vi "LPF.vi"(9 "Cutoff freq":dbl, 10 "Sampling freq":dbl, 11 "x":dbl) -> (2 "y":dbl)   [LabVIEW 2025]
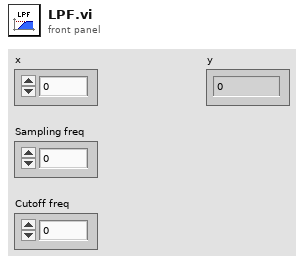
[diagram p1: front panel]
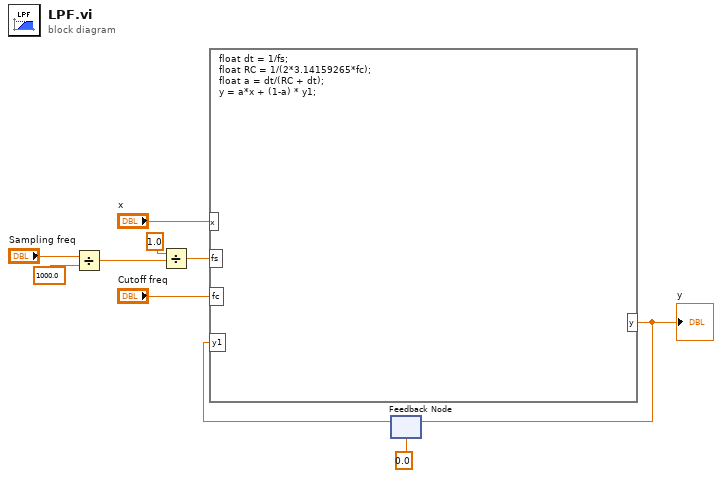
[diagram p0: block diagram]
diagram:
  n1 = Divide(x="Sampling freq", y=1000.0) -> (x/y=w3:dbl)
  n2 = Divide(x=1.0, y=w3) -> (x/y=w5:dbl)
  n3 = feedback #1(0.0 ("y")) -> (w10:dbl)
  n4 = formula code="float dt = 1/fs;\nfloat RC = 1/(2*3.14159265*fc);\nfloat a = dt/(RC + dt);\ny = a*x + (1-a) * y1;"("fs"=w5, "y1"=w10, "fc"="Cutoff freq", "x"="x") -> ("y"=w7:dbl)
  "y" <- w7
  n5 = feedback-in #1(w7) -> ()
